vi "IX83 Device Engine.vi"(0 "Unique Notifier Name":string, 11 "COM Port":string[](array[string])) -> ()   [LabVIEW 2020]
uses:
  Microscopes Type Defs/Microscope Notifier.ctl
  Microscopes Type Defs/Microscope Actions.ctl
  836ca8f3-5aea-47d1-9c98-eb0639b383a2.vi
panel:
  out "Lamp Set Point":dbl
  out "Objective Z Position (um)":dbl
  in  "Lock Base":bool
  out "Last Error":errorcluster
  in  "Quit":bool
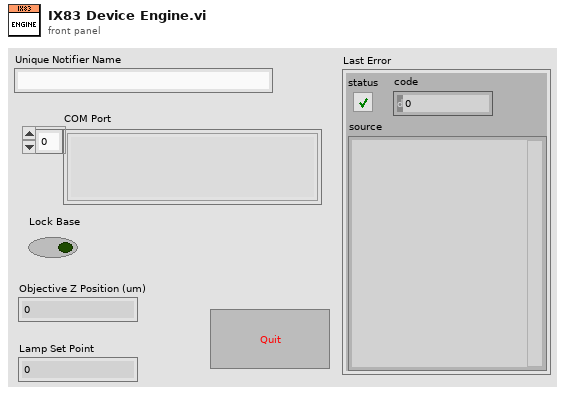
[diagram p1: front panel]
types:
  T1 = typedef "Microscope Actions.ctl" = enum16{"Do Nothing", "Lock Base", "Lock Focus Knob", "Get Objective Index", "Get Objective Z Position", "Get Lamp State", "Get Lamp Power", "Get Output Port", "Get Shutter State", "Get Dichroic Wheel Position", "Set Lamp Index", "Set Shutter Index", "Set Objective Z Position", "Set Lamp State", "Set Lamp Power", "Set Output Port", "Set Shutter State", "Set Dichroic Wheel Position", "Set Objective", "Abort Move", "Set Parameter", "Get Parameter", "Quit"}
  T2 = typedef "Microscope Notifier.ctl" = cluster{"Actions":T1, "Action Done":bool, "Objective Index":u8, "Objective Z Position (um)":dbl, "Lamp Index":u8, "Lamp State":bool, "Output Port":u8, "Shutter Index":u8, "Shutter State":bool, "Dichroic Wheel Position":u8, "Parameter":string, "Parameter Value":string, "Base Locked?":bool, "Obj Speed":u32, "Obj Acceleration":u32, "Obj Deceleration":u32, "Lamp Power (%)":dbl, "Dichroic Wheel Index":u8}
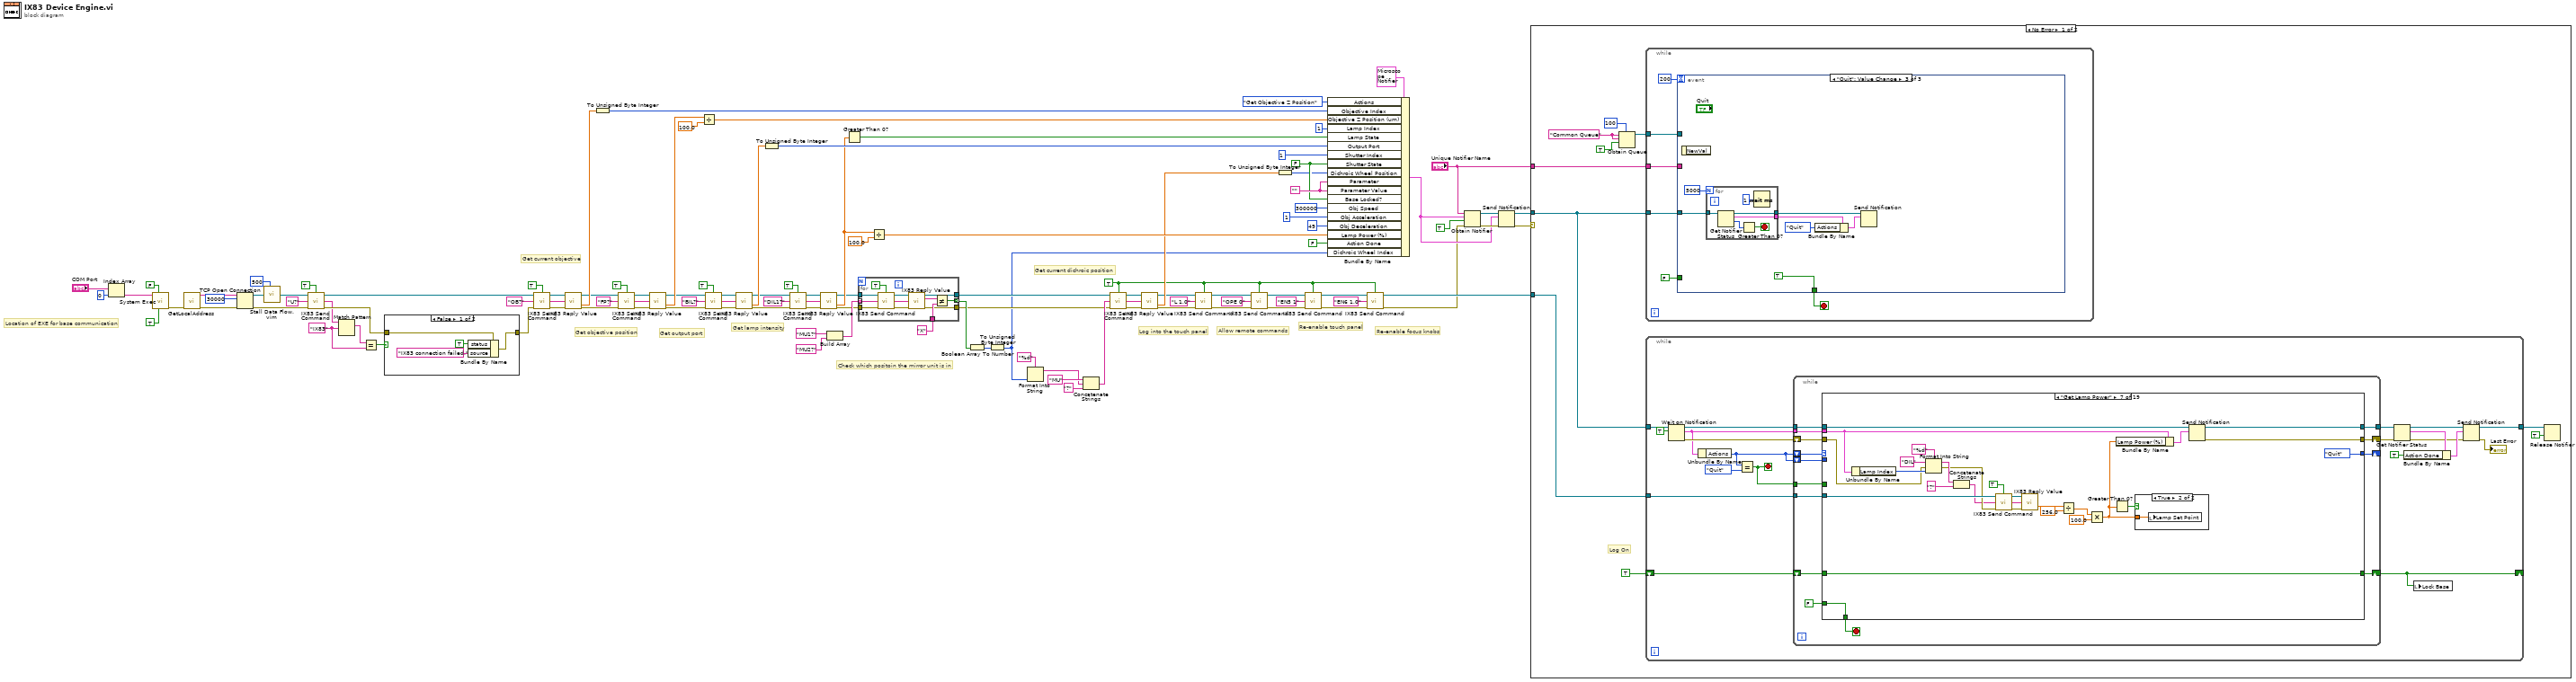
[diagram p0: block diagram]
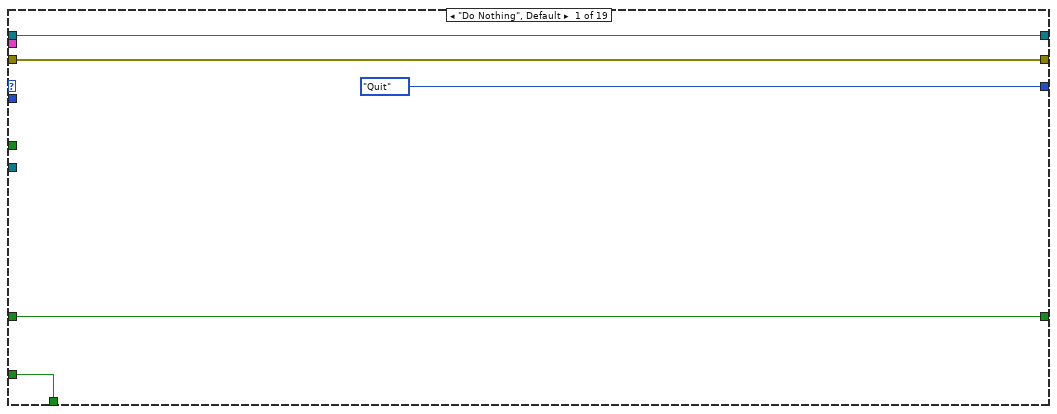
[diagram p2: hidden frame]
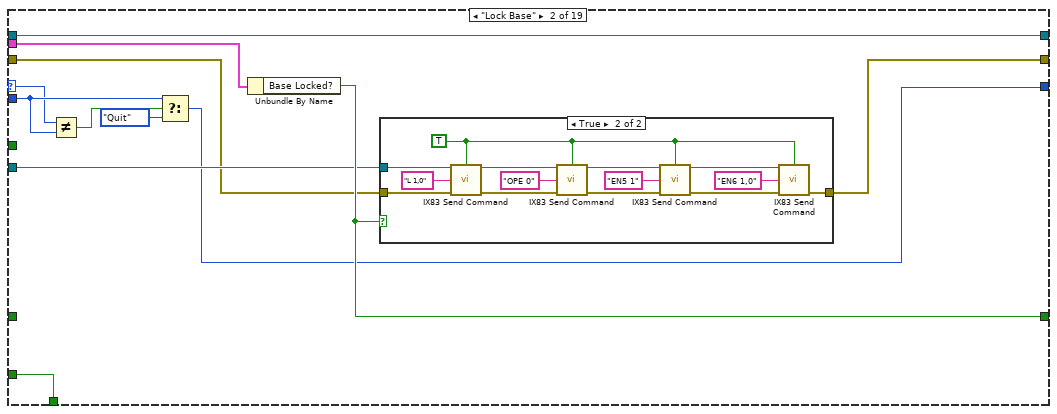
[diagram p3: hidden frame]
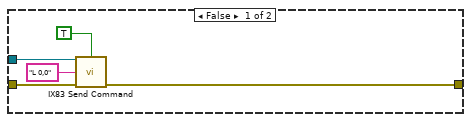
[diagram p4: hidden frame]
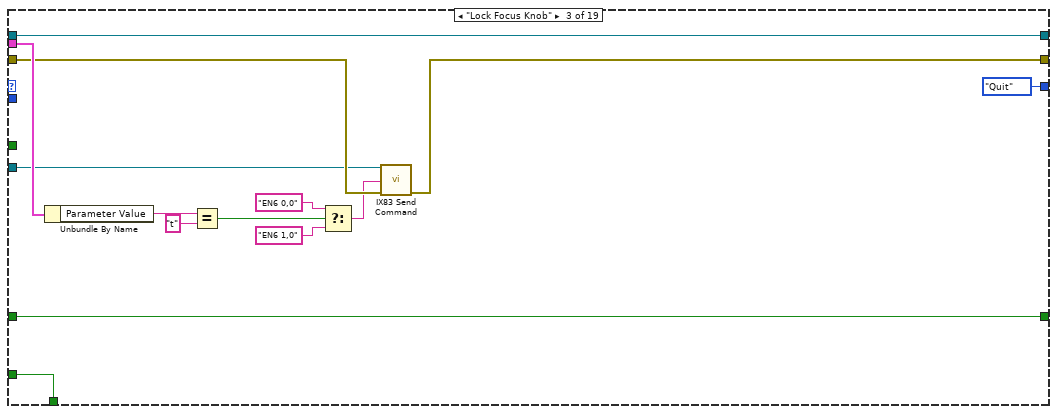
[diagram p5: hidden frame]
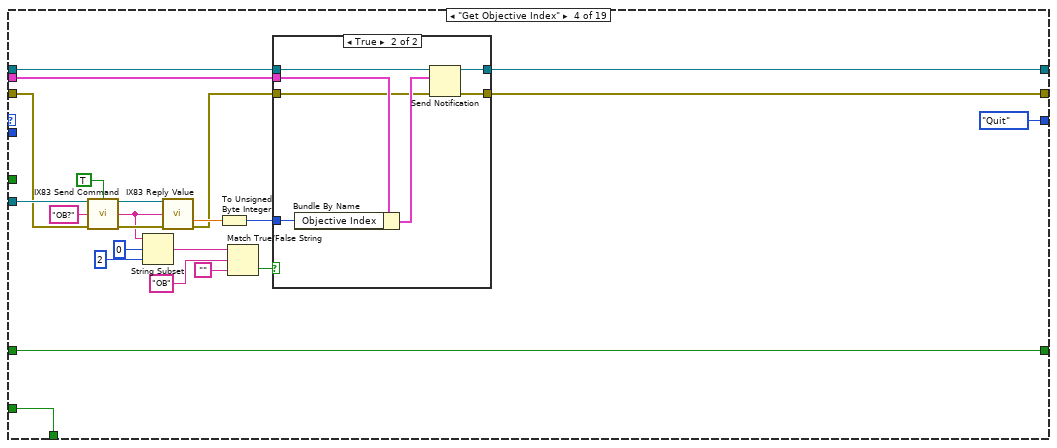
[diagram p6: hidden frame]
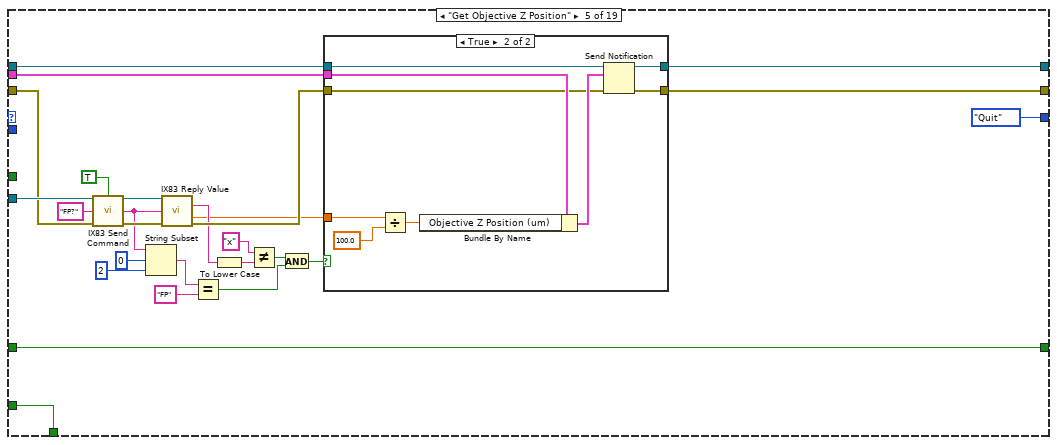
[diagram p8: hidden frame]
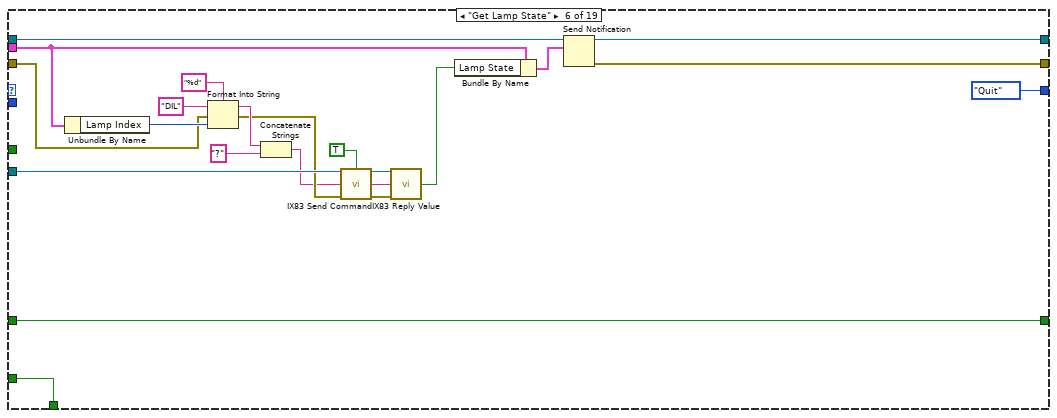
[diagram p10: hidden frame]
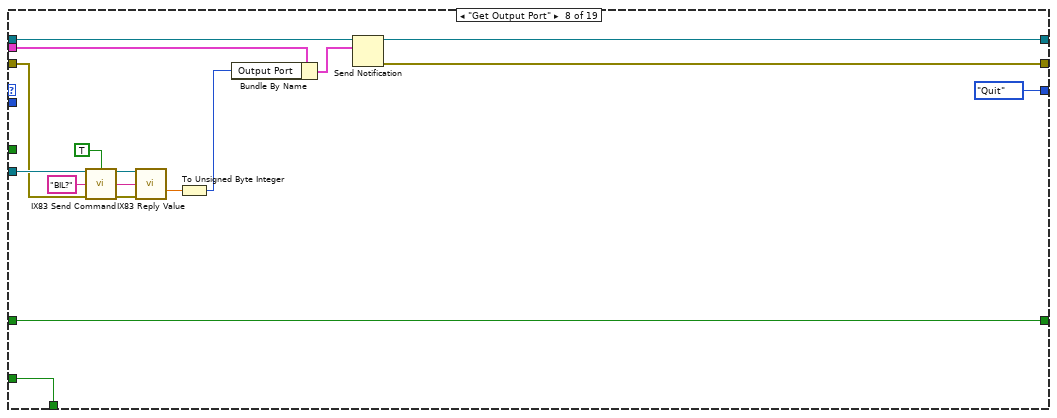
[diagram p12: hidden frame]
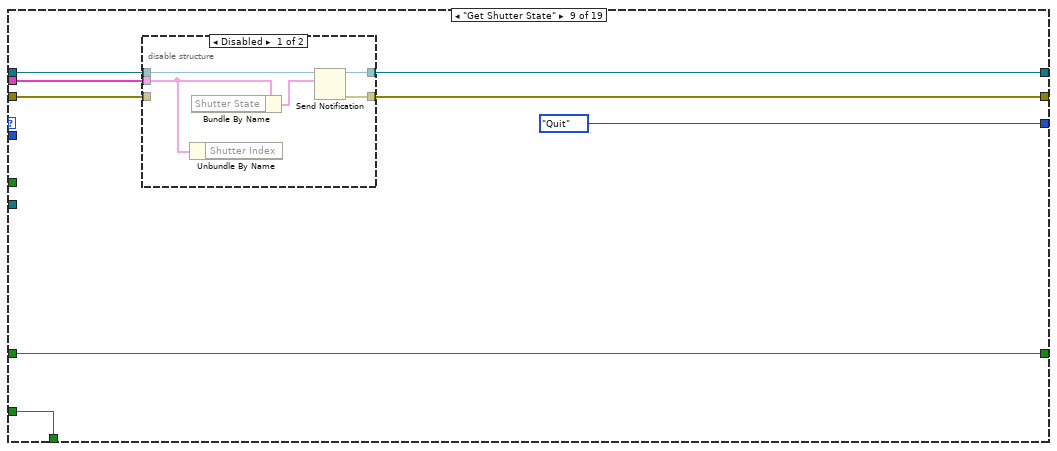
[diagram p13: hidden frame]
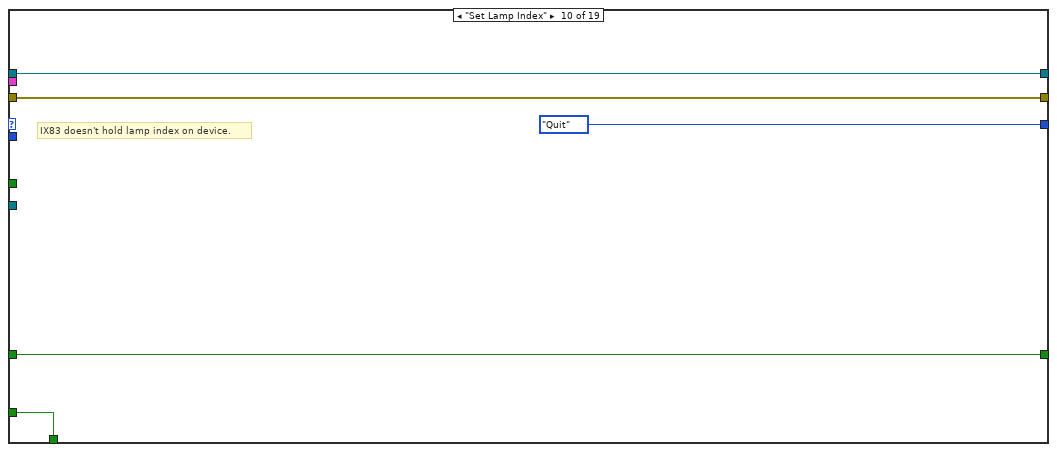
[diagram p15: hidden frame]
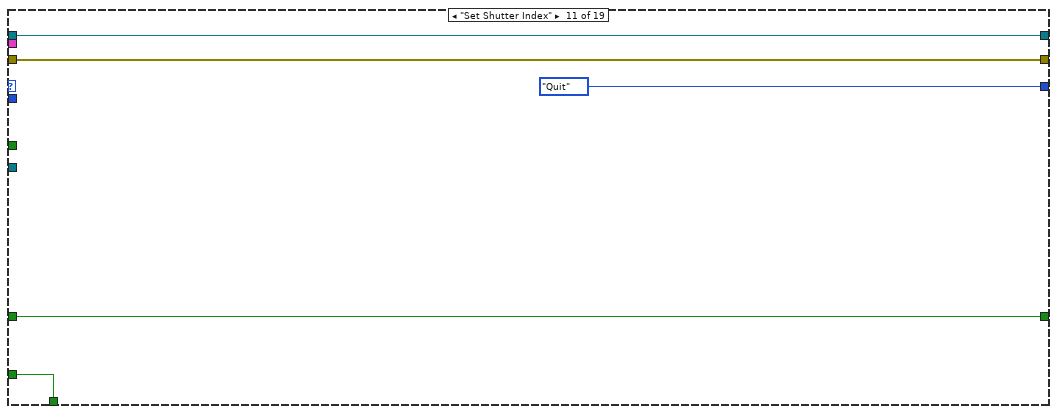
[diagram p16: hidden frame]
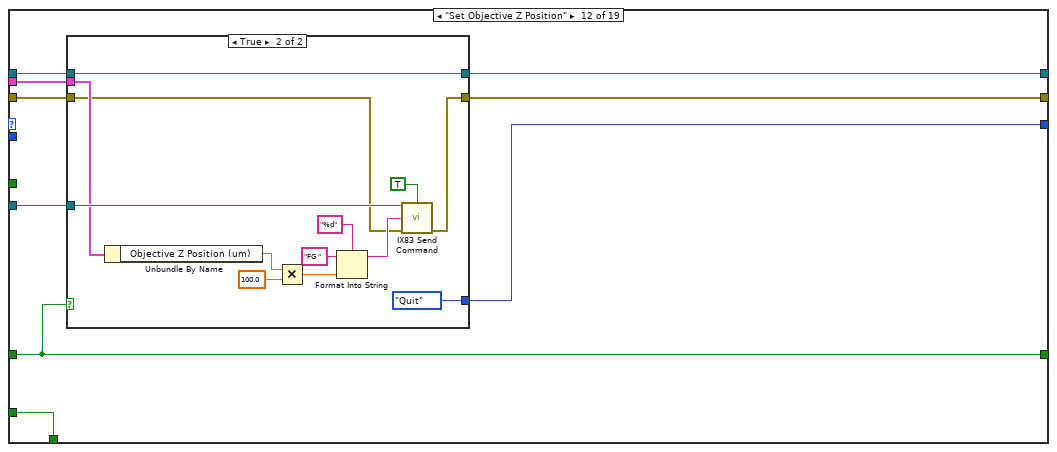
[diagram p17: hidden frame]
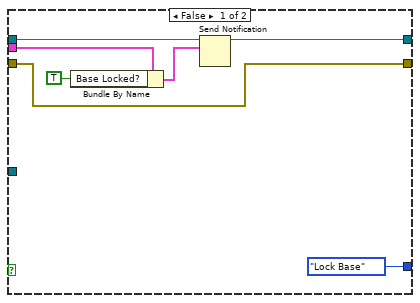
[diagram p18: hidden frame]
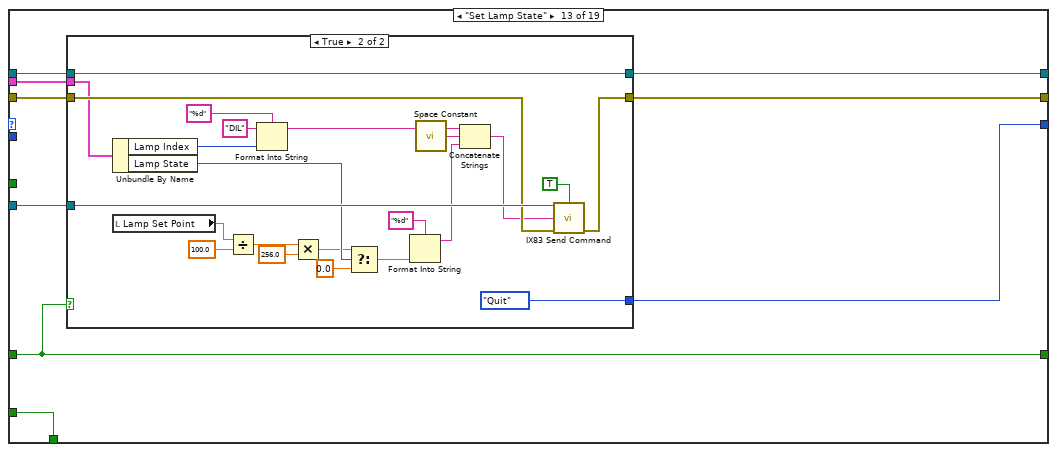
[diagram p19: hidden frame]
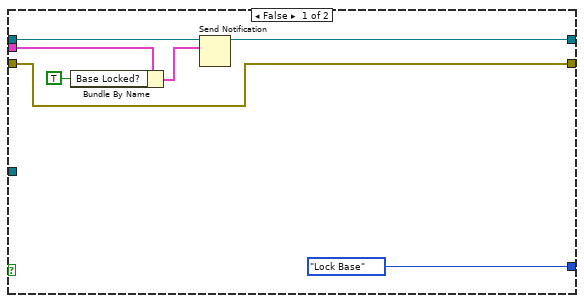
[diagram p20: hidden frame]
diagram:
  w6 = TRUE ("Wait for Reply")
  w86 = "IX83" ("regular expression")
  w100 = FALSE ("Shutter State")
  w108 = ""
  # "Location of EXE for base communication"
  # "Get current dichroic position"
  # "Check which positoin the mirror unit is in"
  # "Get lamp intensity"
  # "Get output port"
  # "Get objective position"
  # "Get current objective"
  # "Re-enable focus knobs"
  # "Re-enable touch panel"
  # "Allow remote commands"
  # "Log into the touch panel"
  n1 = Index Array(array="COM Port", index=0) -> (element=w92:string)
  n2 = call <vilib>:"System Exec.vi"("run minimized? (F)"=TRUE, "wait until completion? (T)"=FALSE, "command line"=w92) -> ("error out"=w90:errorcluster)  [unwired: 5 in, 3 out]
  n3 = call "GetLocalAddress.vi"("Error In"=w90) -> ("IP Address"=w89:string, "Error Out"=w88:errorcluster)  [unwired: 13 in]
  n4 = TCP Open Connection(address=w89, remote port or service name=u16 30000, error in (no error)=w88) -> (connection ID=w85:refnum<k5>, error out=w80:errorcluster)  [unwired: 2 in]
  n5 = call "Stall Data Flow.vim"("value in"=w85, "milliseconds to wait"=u32 500) -> ("value out"=w81:refnum<k5>)  [unwired: 1 out]
  n6 = call "IX83 Send Command.vi"("Connection ID"=w81, "Wait for Reply"=TRUE, "Cmd"="U?" ("data in"), "Error In"=w80) -> ("Connection ID Out"=w75:refnum<k5>, "CMD Reply"=w77:string, "Error Out"=w78:errorcluster)  [unwired: 9 in]
  n7 = Match Pattern(string=w77, regular expression=w86) -> (match substring=w87:string)  [unwired: 1 in, 3 out]
  n8 = Equal?(x=w87, y=w86) -> (x = y?=w83:bool)
  n9 = case shown="False" w83 {
    tunnel: w78 -> [w116 w117]
    tunnel: [w113 w117] -> w73
    frame False {
      n10 = Bundle By Name(cluster=w116, "status"=TRUE, "source"="IX83 connection failed.") -> (w113:errorcluster)
    }
    frame True {
    }
  }
  n11 = call "IX83 Send Command.vi"("Connection ID"=w75, "Wait for Reply"=TRUE, "Cmd"="OB?", "Error In"=w73) -> ("Connection ID Out"=w72:refnum<k5>, "CMD Reply"=w70:string, "Error Out"=w71:errorcluster)  [unwired: 9 in]
  n12 = call "IX83 Reply Value.vi"("Connection ID"=w72, "Reply"=w70, "Error In"=w71) -> ("Connection ID Out"=w62:refnum<k5>, "Value"=w69:dbl, "Error Out"=w61:errorcluster)  [unwired: 8 in, 2 out]
  n13 = To Unsigned Byte Integer(number=w69) -> (unsigned 8bit integer=w68:u8)
  n14 = call "IX83 Send Command.vi"("Connection ID"=w62, "Wait for Reply"=TRUE, "Cmd"="FP?", "Error In"=w61) -> ("Connection ID Out"=w65:refnum<k5>, "CMD Reply"=w67:string, "Error Out"=w66:errorcluster)  [unwired: 9 in]
  n15 = call "IX83 Reply Value.vi"("Connection ID"=w65, "Reply"=w67, "Error In"=w66) -> ("Connection ID Out"=w54:refnum<k5>, "Value"=w60:dbl, "Error Out"=w53:errorcluster)  [unwired: 8 in, 2 out]
  n16 = Divide(x=w60, y=100.0) -> (x/y=w101:dbl)
  n17 = call "IX83 Send Command.vi"("Connection ID"=w54, "Wait for Reply"=TRUE, "Cmd"="BIL?", "Error In"=w53) -> ("Connection ID Out"=w57:refnum<k5>, "CMD Reply"=w55:string, "Error Out"=w56:errorcluster)  [unwired: 9 in]
  n18 = call "IX83 Reply Value.vi"("Connection ID"=w57, "Reply"=w55, "Error In"=w56) -> ("Connection ID Out"=w45:refnum<k5>, "Value"=w52:dbl, "Error Out"=w44:errorcluster)  [unwired: 8 in, 2 out]
  n19 = To Unsigned Byte Integer(number=w52) -> (unsigned 8bit integer=w51:u8)
  n20 = call "IX83 Send Command.vi"("Connection ID"=w45, "Wait for Reply"=TRUE, "Cmd"="DIL1?", "Error In"=w44) -> ("Connection ID Out"=w48:refnum<k5>, "CMD Reply"=w50:string, "Error Out"=w49:errorcluster)  [unwired: 9 in]
  n21 = call "IX83 Reply Value.vi"("Connection ID"=w48, "Reply"=w50, "Error In"=w49) -> ("Connection ID Out"=w35:refnum<k5>, "Value"=w41:dbl, "Error Out"=w34:errorcluster)  [unwired: 8 in, 2 out]
  n22 = Build Array("MU1?" ("Cmd"), "MU2?" ("Cmd")) -> (w36:string[])
  n23 = Greater Than 0?(x=w41) -> (x > 0?=w40:bool)
  n24 = for {
    tunnel: [w125] -> w33 mode=indexing
    tunnel: "X" -> [w124]
    tunnel: w36 -> [w123] mode=indexing
    tunnel: w35 -> [w122]
    tunnel: w34 -> [w121]
    tunnel: [w120] -> w21
    tunnel: [w119] -> w25
    n25 = call "IX83 Send Command.vi"("Connection ID"=w122, "Wait for Reply"=TRUE, "Cmd"=w123, "Error In"=w121) -> ("Connection ID Out"=w128:refnum<k5>, "CMD Reply"=w126:string, "Error Out"=w127:errorcluster)  [unwired: 9 in]
    n26 = call "IX83 Reply Value.vi"("Connection ID"=w128, "Reply"=w126, "Error In"=w127) -> ("Connection ID Out"=w119:refnum<k5>, "Reply"=w118:string, "Error Out"=w120:errorcluster)  [unwired: 8 in, 2 out]
    n27 = Not Equal?(x=w118, y=w124) -> (x != y?=w125:bool)
  }
  n28 = Divide(x=w41, y=100.0) -> (x/y=w42:dbl)
  n29 = Boolean Array To Number(Boolean array=w33) -> (number=w5:u32)
  n30 = To Unsigned Byte Integer(number=w5) -> (unsigned 8bit integer=w4:u8)
  n31 = Format Into String(format string="%d", w4) -> (resulting string=w29:string)  [unwired: 2 in, 1 out]
  n32 = Concatenate Strings("MU", w29, "?" ("string")) -> (w24:string)
  n33 = call "IX83 Send Command.vi"("Connection ID"=w25, "Wait for Reply"=w6, "Cmd"=w24, "Error In"=w21) -> ("Connection ID Out"=w28:refnum<k5>, "CMD Reply"=w26:string, "Error Out"=w27:errorcluster)  [unwired: 9 in]
  n34 = call "IX83 Reply Value.vi"("Connection ID"=w28, "Reply"=w26, "Error In"=w27) -> ("Connection ID Out"=w10:refnum<k5>, "Value"=w23:dbl, "Error Out"=w9:errorcluster)  [unwired: 8 in, 2 out]
  n35 = call "IX83 Send Command.vi"("Connection ID"=w10, "Wait for Reply"=w6, "Cmd"="L 1,0" ("data in"), "Error In"=w9) -> ("Connection ID Out"=w16:refnum<k5>, "Error Out"=w13:errorcluster)  [unwired: 9 in, 1 out]
  n36 = call "IX83 Send Command.vi"("Connection ID"=w16, "Wait for Reply"=w6, "Cmd"="OPE 0" ("data in"), "Error In"=w13) -> ("Connection ID Out"=w15:refnum<k5>, "Error Out"=w12:errorcluster)  [unwired: 9 in, 1 out]
  n37 = To Unsigned Byte Integer(number=w23) -> (unsigned 8bit integer=w22:u8)
  n38 = call "IX83 Send Command.vi"("Connection ID"=w15, "Wait for Reply"=w6, "Cmd"="EN5 1" ("data in"), "Error In"=w12) -> ("Connection ID Out"=w14:refnum<k5>, "Error Out"=w11:errorcluster)  [unwired: 9 in, 1 out]
  n39 = Bundle By Name(cluster=T2 {"Actions"=enum."Get Objective Index", "Action Done"=FALSE, "Objective Index"=0, "Objective Z Position (um)"=0.0, "Lamp Index"=0, "Lamp State"=FALSE, "Output Port"=0, "Shutter Index"=0, "Shutter State"=FALSE, "Dichroic Wheel Position"=0, "Parameter"="", "Parameter Value"="", "Base Locked?"=FALSE, "Obj Speed"=0, "Obj Acceleration"=0, "Obj Deceleration"=0, "Lamp Power (%)"=0.0, "Dichroic Wheel Index"=0} ("Microscope Notifier"), "Actions"=Microscope_Actions."Get Objective Z Position", "Objective Index"=w68, "Objective Z Position (um)"=w101, "Lamp Index"=u8 1, "Lamp State"=w40, "Output Port"=w51, "Shutter Index"=u8 1, "Shutter State"=w100, "Dichroic Wheel Position"=w22, "Parameter"=w108, "Parameter Value"=w108, "Base Locked?"=w100, "Obj Speed"=u32 300000, "Obj Acceleration"=u32 1, "Obj Deceleration"=u32 49, "Lamp Power (%)"=w42, "Action Done"=FALSE, "Dichroic Wheel Index"=w4) -> (w103:T2)
  n40 = call "IX83 Send Command.vi"("Connection ID"=w14, "Wait for Reply"=w6, "Cmd"="EN6 1,0" ("data in"), "Error In"=w11) -> ("Connection ID Out"=w8:refnum<k5>, "Error Out"=w7:errorcluster)  [unwired: 9 in, 1 out]
  n41 = Obtain Notifier(name (unnamed)="Unique Notifier Name", notification data type=w103, create if not found? (T)=TRUE, error in (no error)=w7) -> (notifier out=w107:refnum<notifier>, error out=w105:errorcluster)  [unwired: 1 out]
  n42 = Send Notification(notification=w103, notifier=w107, error in (no error)=w105) -> (notifier out=w106:refnum<notifier>, error out=w104:errorcluster)
  n43 = case shown="No Error" w104 {
    tunnel: "Unique Notifier Name" -> [w135 _]
    tunnel: w106 -> [w130 _]
    tunnel: w8 -> [w132 w586]
    frame No Error {
      w139 = "Common Queue" ("Unique Notifier Name")
      # "Log On"
      n44 = Obtain Queue(max queue size (-1, unlimited)=100, name (unnamed)=w139, element data type=w139, create if not found? (T)=TRUE) -> (queue out=w136:refnum<queue>)  [unwired: 1 in, 2 out]
      n45 = while {
        tunnel: w130 -> [w548]
        tunnel: w136 -> [w545]
        tunnel: w135 -> [w544]
        stop <- w546 stop-if-true
        n46 = event shown="[2] \"Quit\": Value Change" {
          selector: _ -> [_ _ _]
          dyn-events: _ -> [_ _ _]
          timeout: 200 -> [_ _ _]
          tunnel: w548 -> [w562 w567 w576]
          tunnel: [w550 w572 TRUE ("status")] -> w546
          tunnel: w545 -> [w558 _ _]
          tunnel: w544 -> [w557 _ _]
          tunnel: FALSE ("status") -> [_ w572 _]
          event Timeout {
            n47 = event-data() -> ()  [unwired: 1 in, 1 out]
            n48 = Get Notifier Status(notifier=w562) -> (notifier out=w549:refnum<notifier>, current notification=w556:T2, error out=w561:errorcluster)  [unwired: 1 in, 2 out]
            n49 = call "Common Device Queue Get Command.vi"("Common Queue"=w558, "Notifier Name"=w557) -> ("Command"=w560:string)  [unwired: 12 in, 1 out]
            n50 = Unbundle By Name(w561) -> ("status"=w552:bool)
            n51 = control-ref of="This VI"() -> (w559:refnum<vi>)
            n52 = call "Common Device Queue Execute Command.vi"("Common Command"=w560, "VI Refnum"=w559) -> ("Quit?"=w551:bool)  [unwired: 12 in, 1 out]
            n53 = Or(x=w551, y=w552) -> (x .or. y?=w550:bool)
            n54 = case shown="False" w551 {
              tunnel: [Microscope_Actions."Get Objective Z Position" ("Actions") Microscope_Actions."Quit" ("Actions")] -> w553
              frame False {
              }
              frame True {
              }
            }
            n55 = Bundle By Name(cluster=w556, "Actions"=w553) -> (w555:T2)
            n56 = Send Notification(notification=w555, notifier=w549) -> ()  [unwired: 1 in, 2 out]
            n57 = Unbundle By Name(w555) -> ("Objective Z Position (um)"=→"Objective Z Position (um)":dbl)
          }
          event "Lock Base": Value Change {
            n58 = event-data() -> ("NewVal"=w565:bool)  [unwired: 1 in]
            n59 = Get Notifier Status(notifier=w567) -> (notifier out=w570:refnum<notifier>, current notification=w569:T2, error out=w571:errorcluster)  [unwired: 1 in, 2 out]
            n60 = Bundle By Name(cluster=w569, "Actions"=Microscope_Actions."Lock Base", "Base Locked?"=w565) -> (w568:T2)
            n61 = Send Notification(notification=w568, notifier=w570, error in (no error)=w571) -> ()  [unwired: 2 out]
          }
          event "Quit": Value Change {
            n62 = event-data() -> ()  [unwired: 1 in, 1 out]
            n63 = for {
              N: 5000 -> [_]
              tunnel: w576 -> [w585]
              tunnel: [w582] -> w573
              tunnel: [w580] -> w574
              stop <- w583 stop-if-true
              n64 = Get Notifier Status(notifier=w585) -> (notifier out=w582:refnum<notifier>, current notification=w580:T2, # waiting=w584:i32)  [unwired: 1 in, 2 out]
              n65 = Greater Than 0?(x=w584) -> (x > 0?=w583:bool)
              n66 = Wait (ms)(milliseconds to wait=u32 1) -> ()  [unwired: 1 out]
            }
            n67 = Bundle By Name(cluster=w574, "Actions"=Microscope_Actions."Quit") -> (w577:T2)
            n68 = Send Notification(notification=w577, notifier=w573) -> ()  [unwired: 1 in, 2 out]
          }
        }
      }
      n69 = while {
        tunnel: w130 -> [w159]
        tunnel: [w149] -> w134
        tunnel: w132 -> [w156]
        shift-right: [w141] -> _
        shift-left: TRUE -> [w154]
        stop <- w153 stop-if-true
        n70 = Wait on Notification(notifier=w159, ignore previous (F)=TRUE) -> (notifier out=w143:refnum<notifier>, notification=w155:T2, error out=w157:errorcluster)  [unwired: 2 in, 1 out]
        n71 = Unbundle By Name(w155) -> ("Actions"=w140:T1)
        n72 = Equal?(x=w140, y=Microscope_Actions."Quit") -> (x = y?=w153:bool)
        n73 = while {
          shift-right: [w170] -> _
          shift-left: w140 -> [w171]
          tunnel: w143 -> [w168]
          tunnel: [w167] -> w152
          tunnel: w156 -> [w166]
          tunnel: w155 -> [w165]
          shift-right: [w162] -> w141
          shift-left: w154 -> [w163]
          tunnel: w153 -> [w161]
          shift-right: [w164] -> w151
          shift-left: w157 -> [w169]
          shift-left: w140 -> [w160]
          stop <- w172 stop-if-true
          n74 = case shown="\"Get Lamp Power\"" w171 {
            selector: w171 -> [_ w180 _ _ _ _ _ _ _ _ _ _ _ _ _ _ _ _ _]
            tunnel: FALSE -> [w177 w190 w223 w246 w281 w314 w341 w359 w367 w379 w384 w393 w422 w462 w471 w494 w503 w526 _]
            tunnel: [w177 w190 w223 w246 w281 w314 w341 w359 w367 w379 w384 w393 w422 w462 w471 w494 w503 w526 TRUE] -> w172
            tunnel: [Microscope_Actions."Quit" ("y") w179 Microscope_Actions."Quit" ("y") Microscope_Actions."Quit" ("y") Microscope_Actions."Quit" ("y") Microscope_Actions."Quit" ("y") Microscope_Actions."Quit" ("y") Microscope_Actions."Quit" ("y") Microscope_Actions."Quit" ("y") Microscope_Actions."Quit" ("y") Microscope_Actions."Quit" ("y") w390 w419 w453 w465 Microscope_Actions."Quit" ("y") w495 Microscope_Actions."Quit" ("y") Microscope_Actions."Quit" ("y")] -> w170
            tunnel: w169 -> [w175 w185 w213 w227 w265 w301 w328 w346 w360 w375 w381 w386 w415 w459 w469 w490 w501 w522 w529]
            tunnel: w168 -> [w176 w188 w220 w243 w280 w311 w338 w355 w364 w376 w382 w389 w418 w461 w470 w492 w502 w524 w533]
            tunnel: [w176 w188 w220 w242 w279 w310 w337 w354 w363 w376 w382 w387 w416 w461 w464 w492 w497 w524 w533] -> w167
            tunnel: w166 -> [_ w186 w211 w233 w266 w296 w323 w347 _ _ _ w391 w420 _ w466 _ w500 _ w530]
            tunnel: w165 -> [_ w189 w221 w244 w276 w304 w331 w356 w361 _ _ w388 w417 w458 w468 _ w499 _ _]
            tunnel: [w175 w184 w210 w241 w278 w309 w336 w353 w362 w375 w381 w385 w414 w459 w463 w490 w496 w522 w528] -> w164
            tunnel: w163 -> [w174 _ w222 w240 w275 w312 w339 w357 w365 w378 w383 w392 w421 w460 w467 w491 w498 w525 w527]
            tunnel: [w174 w187 w222 w240 w275 w312 w339 w357 w365 w378 w383 w392 w421 w460 w467 w491 w498 w525 w527] -> w162
            tunnel: w161 -> [_ _ _ _ _ _ _ _ _ _ _ _ _ _ _ _ _ _ w531]
            tunnel: w160 -> [_ w181 _ _ _ _ _ _ _ _ _ _ _ _ _ _ _ _ _]
            frame "Do Nothing", Default {
            }
            frame "Lock Base" {
              n75 = Not Equal?(x=w180, y=w181) -> (x != y?=w182:bool)
              n76 = Select(t=w181, s=w182, f=Microscope_Actions."Quit") -> (s? t:f=w179:T1)
              n77 = Unbundle By Name(w189) -> ("Base Locked?"=w187:bool)
              n78 = case shown="True" w187 {
                tunnel: w186 -> [w193 w199]
                tunnel: w185 -> [w192 w198]
                tunnel: [w191 w196] -> w184
                frame False {
                  n79 = call "IX83 Send Command.vi"("Connection ID"=w193, "Wait for Reply"=TRUE, "Cmd"="L 0,0" ("data in"), "Error In"=w192) -> ("Error Out"=w191:errorcluster)  [unwired: 9 in, 2 out]
                }
                frame True {
                  w197 = TRUE ("Wait for Reply")
                  n80 = call "IX83 Send Command.vi"("Connection ID"=w199, "Wait for Reply"=w197, "Cmd"="L 1,0" ("data in"), "Error In"=w198) -> ("Connection ID Out"=w209:refnum<k5>, "Error Out"=w206:errorcluster)  [unwired: 9 in, 1 out]
                  n81 = call "IX83 Send Command.vi"("Connection ID"=w209, "Wait for Reply"=w197, "Cmd"="OPE 0" ("data in"), "Error In"=w206) -> ("Connection ID Out"=w208:refnum<k5>, "Error Out"=w205:errorcluster)  [unwired: 9 in, 1 out]
                  n82 = call "IX83 Send Command.vi"("Connection ID"=w208, "Wait for Reply"=w197, "Cmd"="EN5 1" ("data in"), "Error In"=w205) -> ("Connection ID Out"=w207:refnum<k5>, "Error Out"=w204:errorcluster)  [unwired: 9 in, 1 out]
                  n83 = call "IX83 Send Command.vi"("Connection ID"=w207, "Wait for Reply"=w197, "Cmd"="EN6 1,0" ("data in"), "Error In"=w204) -> ("Error Out"=w196:errorcluster)  [unwired: 9 in, 2 out]
                }
              }
            }
            frame "Lock Focus Knob" {
              n84 = Unbundle By Name(w221) -> ("Parameter Value"=w219:string)
              n85 = Equal?(x=w219, y="t") -> (x = y?=w215:bool)
              n86 = Select(t="EN6 0,0" ("Command"), s=w215, f="EN6 1,0" ("Command")) -> (s? t:f=w212:string)
              n87 = call "IX83 Send Command.vi"("Connection ID"=w211, "Cmd"=w212, "Error In"=w213) -> ("Error Out"=w210:errorcluster)  [unwired: 10 in, 2 out]
            }
            frame "Get Objective Index" {
              n88 = call "IX83 Send Command.vi"("Connection ID"=w233, "Wait for Reply"=TRUE, "Cmd"="OB?", "Error In"=w227) -> ("Connection ID Out"=w231:refnum<k5>, "CMD Reply"=w229:string, "Error Out"=w230:errorcluster)  [unwired: 9 in]
              n89 = String Subset(string=w229, offset (0)=0, length (rest)=2 ("length (rest)")) -> (substring=w237:string)
              n90 = call "IX83 Reply Value.vi"("Connection ID"=w231, "Reply"=w229, "Error In"=w230) -> ("Value"=w228:dbl, "Error Out"=w226:errorcluster)  [unwired: 8 in, 3 out]
              n91 = To Unsigned Byte Integer(number=w228) -> (unsigned 8bit integer=w225:u8)
              n92 = Match True/False String(2:"", 3:"OB" ("regular expression"), 4:w237) -> (0:w234:bool)  [unwired: 1 out]
              n93 = case shown="True" w234 {
                tunnel: w244 -> [_ w255]
                tunnel: w243 -> [w248 w254]
                tunnel: [w248 w253] -> w242
                tunnel: w226 -> [w247 w251]
                tunnel: [w247 w250] -> w241
                tunnel: w225 -> [_ w249]
                frame False {
                }
                frame True {
                  n94 = Bundle By Name(cluster=w255, "Objective Index"=w249) -> (w252:T2)
                  n95 = Send Notification(notification=w252, notifier=w254, error in (no error)=w251) -> (notifier out=w253:refnum<notifier>, error out=w250:errorcluster)
                }
              }
            }
            frame "Get Objective Z Position" {
              n96 = call "IX83 Send Command.vi"("Connection ID"=w266, "Wait for Reply"=TRUE, "Cmd"="FP?", "Error In"=w265) -> ("Connection ID Out"=w269:refnum<k5>, "CMD Reply"=w263:string, "Error Out"=w270:errorcluster)  [unwired: 9 in]
              n97 = String Subset(string=w263, offset (0)=0, length (rest)=2 ("length (rest)")) -> (substring=w272:string)
              n98 = call "IX83 Reply Value.vi"("Connection ID"=w269, "Reply"=w263, "Error In"=w270) -> ("Reply"=w262:string, "Value"=w256:dbl, "Error Out"=w264:errorcluster)  [unwired: 8 in, 2 out]
              n99 = Equal?(x=w272, y="FP") -> (x = y?=w258:bool)
              n100 = To Lower Case(string=w262) -> (all lower case string=w261:string)
              n101 = Not Equal?(x="x", y=w261) -> (x != y?=w259:bool)
              n102 = And(x=w259, y=w258) -> (x .and. y?=w257:bool)
              n103 = case shown="True" w257 {
                tunnel: w280 -> [w283 w291]
                tunnel: [w283 w290] -> w279
                tunnel: [w282 w289] -> w278
                tunnel: w276 -> [_ w288]
                tunnel: w264 -> [w282 w285]
                tunnel: w256 -> [_ w284]
                frame False {
                }
                frame True {
                  n104 = Divide(x=w284, y=100.0) -> (x/y=w287:dbl)
                  n105 = Bundle By Name(cluster=w288, "Objective Z Position (um)"=w287) -> (w286:T2)
                  n106 = Send Notification(notification=w286, notifier=w291, error in (no error)=w285) -> (notifier out=w290:refnum<notifier>, error out=w289:errorcluster)
                }
              }
            }
            frame "Get Lamp State" {
              n107 = Unbundle By Name(w304) -> ("Lamp Index"=w303:u8)
              n108 = Format Into String(format string="%d", initial string="DIL" ("Cmd"), error in=w301, w303) -> (resulting string=w302:string, error out=w295:errorcluster)
              n109 = Concatenate Strings(w302, "?" ("Cmd")) -> (w294:string)
              n110 = call "IX83 Send Command.vi"("Connection ID"=w296, "Wait for Reply"=TRUE, "Cmd"=w294, "Error In"=w295) -> ("Connection ID Out"=w299:refnum<k5>, "CMD Reply"=w298:string, "Error Out"=w300:errorcluster)  [unwired: 9 in]
              n111 = call "IX83 Reply Value.vi"("Connection ID"=w299, "Reply"=w298, "Error In"=w300) -> ("Bool"=w293:bool)  [unwired: 8 in, 4 out]
              n112 = Bundle By Name(cluster=w304, "Lamp State"=w293) -> (w308:T2)
              n113 = Send Notification(notification=w308, notifier=w311) -> (notifier out=w310:refnum<notifier>, error out=w309:errorcluster)  [unwired: 1 in]
            }
            frame "Get Lamp Power" {
              n114 = Unbundle By Name(w331) -> ("Lamp Index"=w330:u8)
              n115 = Format Into String(format string="%d", initial string="DIL" ("Cmd"), error in=w328, w330) -> (resulting string=w329:string, error out=w322:errorcluster)
              n116 = Concatenate Strings(w329, "?" ("Cmd")) -> (w321:string)
              n117 = call "IX83 Send Command.vi"("Connection ID"=w323, "Wait for Reply"=TRUE, "Cmd"=w321, "Error In"=w322) -> ("Connection ID Out"=w326:refnum<k5>, "CMD Reply"=w325:string, "Error Out"=w327:errorcluster)  [unwired: 9 in]
              n118 = call "IX83 Reply Value.vi"("Connection ID"=w326, "Reply"=w325, "Error In"=w327) -> ("Value"=w320:dbl)  [unwired: 8 in, 4 out]
              n119 = Divide(x=w320, y=256.0) -> (x/y=w318:dbl)
              n120 = Multiply(x=w318, y=100.0) -> (x*y=w315:dbl)
              n121 = Greater Than 0?(x=w315) -> (x > 0?=w316:bool)
              n122 = Bundle By Name(cluster=w331, "Lamp Power (%)"=w315) -> (w335:T2)
              n123 = case shown="True" w316 {
                tunnel: w315 -> [_ w342]
                frame False {
                }
                frame True {
                  n124 = local write "Lamp Set Point"(w342) -> ()
                }
              }
              n125 = Send Notification(notification=w335, notifier=w338) -> (notifier out=w337:refnum<notifier>, error out=w336:errorcluster)  [unwired: 1 in]
            }
            frame "Get Output Port" {
              n126 = call "IX83 Send Command.vi"("Connection ID"=w347, "Wait for Reply"=TRUE, "Cmd"="BIL?", "Error In"=w346) -> ("Connection ID Out"=w350:refnum<k5>, "CMD Reply"=w349:string, "Error Out"=w351:errorcluster)  [unwired: 9 in]
              n127 = call "IX83 Reply Value.vi"("Connection ID"=w350, "Reply"=w349, "Error In"=w351) -> ("Value"=w344:dbl)  [unwired: 8 in, 4 out]
              n128 = To Unsigned Byte Integer(number=w344) -> (unsigned 8bit integer=w343:u8)
              n129 = Bundle By Name(cluster=w356, "Output Port"=w343) -> (w352:T2)
              n130 = Send Notification(notification=w352, notifier=w355) -> (notifier out=w354:refnum<notifier>, error out=w353:errorcluster)  [unwired: 1 in]
            }
            frame "Get Shutter State" {
              n131 = disable-structure shown="Disabled" {
                disable-tunnel: w364 -> [w372 w374]
                disable-tunnel: [w371 w374] -> w363
                disable-tunnel: [w369 w373] -> w362
                disable-tunnel: w361 -> [w368 _]
                disable-tunnel: w360 -> [_ w373]
                frame Disabled {
                  n132 = Unbundle By Name(w368) -> ()  [unwired: 1 out]
                  n133 = Bundle By Name(cluster=w368) -> (w370:T2)  [unwired: 1 in]
                  n134 = Send Notification(notification=w370, notifier=w372) -> (notifier out=w371:refnum<notifier>, error out=w369:errorcluster)  [unwired: 1 in]
                }
                frame Enabled {
                }
              }
            }
            frame "Set Lamp Index" {
              # "IX83 doesn't hold lamp index on device."
            }
            frame "Set Shutter Index" {
            }
            frame "Set Objective Z Position" {
              n135 = case shown="True" w392 {
                tunnel: w391 -> [_ w412]
                tunnel: [Microscope_Actions."Lock Base" ("y") Microscope_Actions."Quit" ("y")] -> w390
                tunnel: w389 -> [w398 w401]
                tunnel: w388 -> [w397 w404]
                tunnel: [w395 w401] -> w387
                tunnel: w386 -> [w394 w403]
                tunnel: [w394 w402] -> w385
                frame False {
                  n136 = Bundle By Name(cluster=w397, "Base Locked?"=TRUE) -> (w399:T2)
                  n137 = Send Notification(notification=w399, notifier=w398) -> (notifier out=w395:refnum<notifier>)  [unwired: 1 in, 1 out]
                }
                frame True {
                  n138 = Unbundle By Name(w404) -> ("Objective Z Position (um)"=w411:dbl)
                  n139 = Multiply(x=w411, y=100.0) -> (x*y=w409:dbl)
                  n140 = Format Into String(format string="%d", initial string="FG ", w409) -> (resulting string=w406:string)  [unwired: 1 in, 1 out]
                  n141 = call "IX83 Send Command.vi"("Connection ID"=w412, "Wait for Reply"=TRUE, "Cmd"=w406, "Error In"=w403) -> ("Error Out"=w402:errorcluster)  [unwired: 9 in, 2 out]
                }
              }
            }
            frame "Set Lamp State" {
              n142 = case shown="True" w421 {
                tunnel: w420 -> [_ w451]
                tunnel: [Microscope_Actions."Lock Base" ("y") Microscope_Actions."Quit" ("y")] -> w419
                tunnel: w418 -> [w427 w446]
                tunnel: w417 -> [w426 w445]
                tunnel: [w424 w446] -> w416
                tunnel: w415 -> [w423 w448]
                tunnel: [w423 w447] -> w414
                frame False {
                  n143 = Bundle By Name(cluster=w426, "Base Locked?"=TRUE) -> (w428:T2)
                  n144 = Send Notification(notification=w428, notifier=w427) -> (notifier out=w424:refnum<notifier>)  [unwired: 1 in, 1 out]
                }
                frame True {
                  n145 = Unbundle By Name(w445) -> ("Lamp Index"=w444:u8, "Lamp State"=w438:bool)
                  n146 = local read "Lamp Set Point"() -> (w430:dbl)
                  n147 = Divide(x=w430, y=100.0) -> (x/y=w440:dbl)
                  n148 = Format Into String(format string="%d", initial string="DIL", w444) -> (resulting string=w434:string)  [unwired: 1 in, 1 out]
                  n149 = Multiply(x=w440, y=256.0) -> (x*y=w437:dbl)
                  n150 = Select(t=w437, s=w438, f=0.0) -> (s? t:f=w435:dbl)
                  n151 = Format Into String(format string="%d", w435) -> (resulting string=w432:string)  [unwired: 2 in, 1 out]
                  n152 = call <vilib>:"Space Constant.vi"() -> ("String"=w433:string)
                  n153 = Concatenate Strings(w434, w433, w432) -> (w431:string)
                  n154 = call "IX83 Send Command.vi"("Connection ID"=w451, "Wait for Reply"=TRUE, "Cmd"=w431, "Error In"=w448) -> ("Error Out"=w447:errorcluster)  [unwired: 9 in, 2 out]
                }
              }
            }
            frame "Set Lamp Power" {
              n155 = Unbundle By Name(w458) -> ("Lamp Power (%)"=→"Lamp Set Point":dbl, "Lamp State"=w456:bool)
              n156 = Select(t=Microscope_Actions."Set Lamp State" ("y"), s=w456, f=Microscope_Actions."Quit" ("y")) -> (s? t:f=w453:T1)
            }
            frame "Set Output Port" {
              n157 = case shown="True" w467 {
                tunnel: w466 -> [_ w488]
                tunnel: [Microscope_Actions."Lock Base" ("y") Microscope_Actions."Quit" ("y")] -> w465
                tunnel: w470 -> [w476 w483]
                tunnel: w468 -> [w475 w482]
                tunnel: [w473 w483] -> w464
                tunnel: w469 -> [w472 w485]
                tunnel: [w472 w484] -> w463
                frame False {
                  n158 = Bundle By Name(cluster=w475, "Base Locked?"=TRUE) -> (w477:T2)
                  n159 = Send Notification(notification=w477, notifier=w476) -> (notifier out=w473:refnum<notifier>)  [unwired: 1 in, 1 out]
                }
                frame True {
                  n160 = Unbundle By Name(w482) -> ("Output Port"=w481:u8)
                  n161 = Format Into String(format string="%d", initial string="BIL ", w481) -> (resulting string=w479:string)  [unwired: 1 in, 1 out]
                  n162 = call "IX83 Send Command.vi"("Connection ID"=w488, "Wait for Reply"=TRUE, "Cmd"=w479, "Error In"=w485) -> ("Error Out"=w484:errorcluster)  [unwired: 9 in, 2 out]
                }
              }
            }
            frame "Set Shutter State" {
            }
            frame "Set Objective" {
              n163 = case shown="True" w498 {
                tunnel: w500 -> [_ w520]
                tunnel: [Microscope_Actions."Lock Base" ("y") Microscope_Actions."Quit" ("y")] -> w495
                tunnel: w502 -> [w508 w515]
                tunnel: w499 -> [w507 w514]
                tunnel: [w505 w515] -> w497
                tunnel: w501 -> [w504 w517]
                tunnel: [w504 w516] -> w496
                frame False {
                  n164 = Bundle By Name(cluster=w507, "Base Locked?"=TRUE) -> (w509:T2)
                  n165 = Send Notification(notification=w509, notifier=w508) -> (notifier out=w505:refnum<notifier>)  [unwired: 1 in, 1 out]
                }
                frame True {
                  n166 = Unbundle By Name(w514) -> ("Objective Index"=w513:u8)  [unwired: 1 out]
                  n167 = Format Into String(format string="%d", initial string="OB ", w513) -> (resulting string=w511:string)  [unwired: 1 in, 1 out]
                  n168 = call "IX83 Send Command.vi"("Connection ID"=w520, "Wait for Reply"=TRUE, "Cmd"=w511, "Error In"=w517) -> ("Error Out"=w516:errorcluster)  [unwired: 9 in, 2 out]
                }
              }
            }
            frame "Abort Move" {
            }
            frame "Quit" {
              n169 = case shown="True" w531 {
                tunnel: w530 -> [_ w540]
                tunnel: w529 -> [w535 w539]
                tunnel: [w535 w536] -> w528
                frame False {
                }
                frame True {
                  n170 = call "IX83 Send Command.vi"("Connection ID"=w540, "Wait for Reply"=TRUE, "Cmd"="L 0,0", "Error In"=w539) -> ("Connection ID Out"=w537:refnum<k5>, "Error Out"=w538:errorcluster)  [unwired: 9 in, 1 out]
                  n171 = TCP Close Connection(connection ID=w537, error in (no error)=w538) -> (error out=w536:errorcluster)  [unwired: 1 in, 1 out]
                }
              }
            }
          }
        }
        n172 = Get Notifier Status(notifier=w152, error in (no error)=w151) -> (notifier out=w150:refnum<notifier>, current notification=w148:T2, error out=w144:errorcluster)  [unwired: 2 out]
        n173 = Bundle By Name(cluster=w148, "Action Done"=TRUE) -> (w146:T2)
        n174 = local write "Lock Base"(w141) -> ()
        n175 = Send Notification(notification=w146, notifier=w150, error in (no error)=w144) -> (notifier out=w149:refnum<notifier>, error out=→"Last Error":errorcluster)
      }
      n176 = Release Notifier(notifier=w134, force destroy? (F)=TRUE) -> ()  [unwired: 1 in, 3 out]
    }
    frame Error {
      n177 = TCP Close Connection(connection ID=w586) -> ()  [unwired: 2 in, 2 out]
    }
  }
